vi "motor step.vi"(8 "error in (no error)":errorcluster, 9 "direction":enum16{"counter-clockwise", "clockwise"}(ring), 10 "steps":i32=1, 11 "Handle In":i32) -> (0 "error out":errorcluster, 1 "Error state":bool, 2 "steps performed":i32, 3 "Handle Out":i32)   [LabVIEW 2013]
uses:
  motor global state actions.ctl
  motor constants.ctl
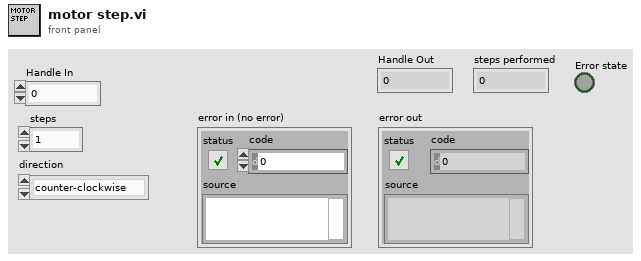
[diagram p1: front panel]
types:
  T1 = typedef "motor global state actions.ctl" = enum16{"set value", "get value", "set angle", "set initialized", "set complete", "set handle", "get handle"}
  T2 = typedef "motor constants.ctl" = u16
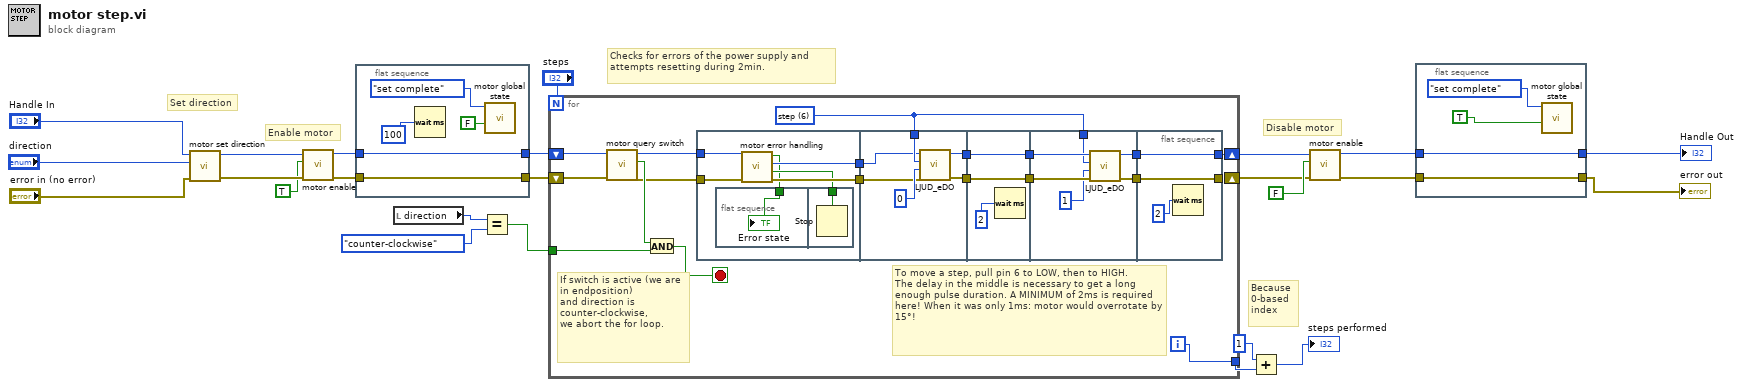
[diagram p0: block diagram]
diagram:
  # "Checks for errors of the power supply and attempts resetting during 2min."
  # "Because \n0-based \nindex"
  # "Disable motor"
  # "Enable motor"
  # "Set direction"
  n1 = call "motor set direction.vi"("error in (no error)"="error in (no error)", "direction"="direction", "Handle In"="Handle In") -> ("error out"=w11:errorcluster, "Handle Out"=w10:i32)  [unwired: 7 in]
  n2 = call "motor enable.vi"("error in (no error)"=w11, "enable"=TRUE, "Handle In"=w10) -> ("error out"=w13:errorcluster, "Handle Out"=w12:i32)  [unwired: 7 in]
  n3 = flat-sequence {
    tunnel: w12 -> [w28]
    tunnel: w13 -> [w29]
    tunnel: [w29] -> w20
    tunnel: [w28] -> w19
    frame #0 {
      n4 = Wait (ms)(milliseconds to wait=100) -> ()  [unwired: 1 out]
      n5 = call "motor global state.vi"("completed"=FALSE, "action"=motor_global_state_actions."set complete" ("Motor FGV actions")) -> ()  [unwired: 8 in, 2 out]
    }
  }
  n6 = local read "direction"() -> (w23:enum16{"counter-clockwise", "clockwise"})
  n7 = Equal?(x=w23, y=enum16{"counter-clockwise", "clockwise"}."counter-clockwise" ("direction")) -> (x = y?=w21:bool)
  n8 = for {
    N: "steps" -> [_]
    tunnel: w21 -> [w37]
    tunnel: [w39] -> w3
    shift-right: [w47] -> w6
    shift-left: w19 -> [w36]
    shift-right: [w48] -> w7
    shift-left: w20 -> [w35]
    i -> [w39]
    stop <- w38 stop-if-true
    w41 = T2 6 items=["enable"=4, "direction"=5, "step"=6, "end switch"=7] ("motor pin settings")
    # "To move a step, pull pin 6 to LOW, then to HIGH.\nThe delay in the middle is necessary to get a long enough pulse duration. A MINIMUM of 2ms is required here! When it was only 1ms: motor would overrotate by 15°!"
    # "If switch is active (we are in endposition)\nand direction is counter-clockwise,\nwe abort the for loop."
    n9 = call "motor query switch.vi"("error in (no error)"=w35, "Handle In"=w36) -> ("error out"=w30:errorcluster, "switch state"=w34:bool, "Handle Out"=w33:i32)  [unwired: 7 in]
    n10 = And(x=w34, y=w37) -> (x .and. y?=w38:bool)
    n11 = flat-sequence {
      tunnel: w33 -> [w54]
      tunnel: [w53] -> w32
      tunnel: [w52] -> w31
      tunnel: w30 -> [w51]
      tunnel: w41 -> [w62]
      tunnel: [w59] -> w43
      tunnel: [w60] -> w40
      tunnel: w32 -> [w58]
      tunnel: w31 -> [w57]
      tunnel: [w65] -> w44
      tunnel: w43 -> [w64]
      tunnel: [w64] -> w42
      tunnel: w40 -> [w65]
      tunnel: w44 -> [w71]
      tunnel: [w68] -> w46
      tunnel: w42 -> [w70]
      tunnel: [w69] -> w45
      tunnel: w41 -> [w66]
      tunnel: [w74] -> w48
      tunnel: w46 -> [w74]
      tunnel: [w73] -> w47
      tunnel: w45 -> [w73]
      frame #0 {
        n12 = flat-sequence {
          tunnel: w49 -> [w55]
          tunnel: w50 -> [w56]
          frame #0 {
            "Error state" <- w55
          }
          frame #1 {
            n13 = Stop(stop? (T)=w56) -> ()
          }
        }
        n14 = call "motor error handling.vi"("error in (no error)"=w51, "Handle in"=w54) -> ("error out"=w52:errorcluster, "Stop .vi?"=w50:bool, "Handle Out out"=w53:i32, "Error state"=w49:bool)  [unwired: 6 in]
      }
      frame #1 {
        n15 = call <vilib>:"LJUD_eDO.vi"("error in"=w57, "State"=0, "Channel"=w62, "Handle In"=w58) -> ("error out"=w60:errorcluster, "Handle Out"=w59:i32)  [unwired: 6 in]
      }
      frame #2 {
        n16 = Wait (ms)(milliseconds to wait=2) -> ()  [unwired: 1 out]
      }
      frame #3 {
        n17 = call <vilib>:"LJUD_eDO.vi"("error in"=w71, "State"=1, "Channel"=w66, "Handle In"=w70) -> ("error out"=w68:errorcluster, "Handle Out"=w69:i32)  [unwired: 6 in]
      }
      frame #4 {
        n18 = Wait (ms)(milliseconds to wait=2) -> ()  [unwired: 1 out]
      }
    }
  }
  n19 = Add(x=1, y=w3) -> (x+y=→"steps performed":i32)
  n20 = call "motor enable.vi"("error in (no error)"=w7, "enable"=FALSE, "Handle In"=w6) -> ("error out"=w5:errorcluster, "Handle Out"=w4:i32)  [unwired: 7 in]
  n21 = flat-sequence {
    tunnel: w4 -> [w77]
    tunnel: w5 -> [w78]
    tunnel: [w78] -> w18
    tunnel: [w77] -> w17
    frame #0 {
      n22 = call "motor global state.vi"("completed"=TRUE, "action"=motor_global_state_actions."set complete" ("Motor FGV actions")) -> ()  [unwired: 8 in, 2 out]
    }
  }
  "Handle Out" <- w17
  "error out" <- w18
